vi "test-0mq.vi"() -> ()   [LabVIEW 2020]
uses:
  <vilib>/addons/zeromq/socket_type.ctl
  <vilib>/addons/zeromq/zmq_context.lvclass
  <vilib>/addons/zeromq/zeromq.lvlib
  <vilib>/addons/zeromq/zmq_socket.lvclass
panel:
  out "?":string
  in  "stop":bool
  out "error out":errorcluster
  out "data":string
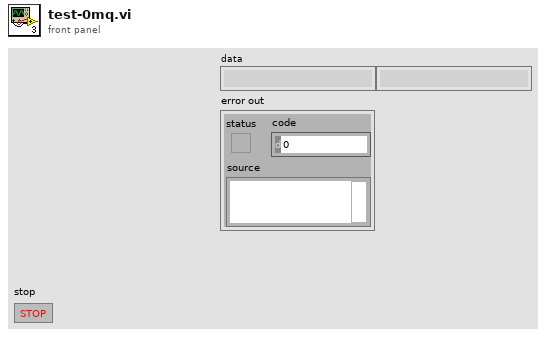
[diagram p1: front panel]
types:
  T1 = typedef "zeromq.lvlib/socket_type.ctl" = enum8{"ZMQ_PAIR", "ZMQ_PUB", "ZMQ_SUB", "ZMQ_REQ", "ZMQ_REP", "ZMQ_DEALER", "ZMQ_ROUTER", "ZMQ_PULL", "ZMQ_PUSH", "ZMQ_XPUB", "ZMQ_XSUB", "ZMQ_STREAM", "ZMQ_SERVER", "ZMQ_CLIENT", "ZMQ_RADIO", "ZMQ_DISH", "ZMQ_GATHER", "ZMQ_SCATTER", "ZMQ_DGRAM"}
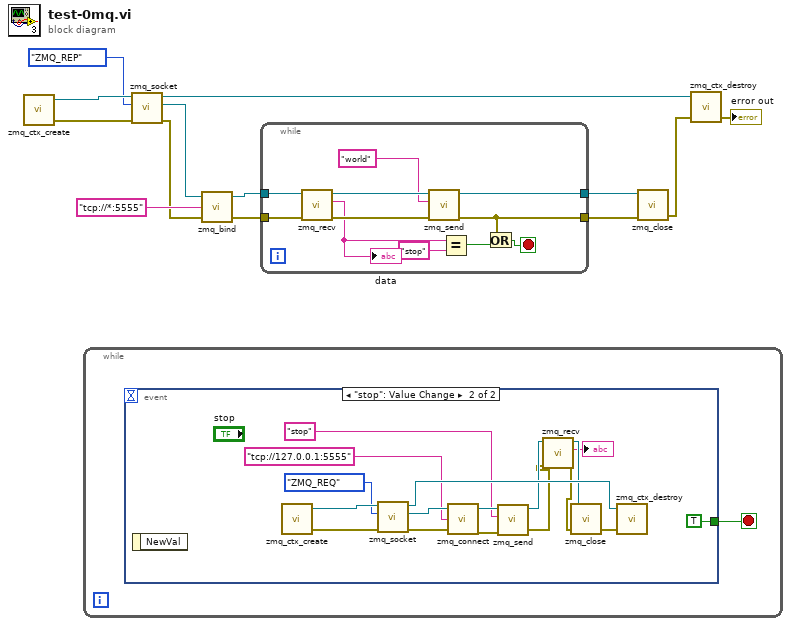
[diagram p0: block diagram]
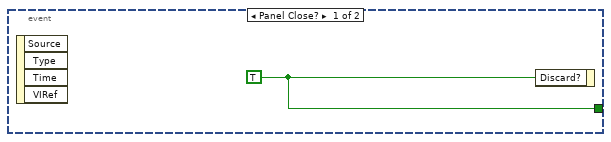
[diagram p2: hidden frame]
diagram:
  n1 = call <vilib>:"zmq_ctx_create.vi"() -> ("error out"=w12:errorcluster, "context out"=w13:refnum<class "zmq_context.lvclass">)  [unwired: 4 in]
  n2 = while {
    stop <- w14 stop-if-true
    n3 = event shown="[1] \"stop\": Value Change" {
      selector: _ -> [_ _]
      dyn-events: _ -> [_ _]
      timeout: _ -> [_ _]
      tunnel: [w15 TRUE] -> w14
      event Panel Close? {
        w15 = TRUE
        n4 = event-data() -> ()  [unwired: 1 in, 4 out]
        n5 = event-data("Discard?"=w15) -> ()  [unwired: 1 in, 1 out]
      }
      event "stop": Value Change {
        n6 = event-data() -> ()  [unwired: 1 in, 1 out]
        n7 = call <vilib>:"zmq_ctx_create.vi"() -> ("error out"=w26:errorcluster, "context out"=w25:refnum<class "zmq_context.lvclass">)  [unwired: 4 in]
        n8 = call <vilib>:"zmq_socket.vi"("error in"=w26, "socket type"=socket_type."ZMQ_REQ", "context in"=w25) -> ("error out"=w28:errorcluster, "socket out"=w27:refnum<class "zmq_socket.lvclass">, "context out"=w32:refnum<class "zmq_context.lvclass">)  [unwired: 2 in]
        n9 = call <vilib>:"zmq_connect.vi"("error in"=w28, "endpoint"="tcp://127.0.0.1:5555", "socket in"=w27) -> ("error out"=w30:errorcluster, "socket out"=w29:refnum<class "zmq_socket.lvclass">)  [unwired: 1 in]
        n10 = call <vilib>:"zmq_send.vi"("error in"=w30, "data"="stop", "socket in"=w29) -> ("error out"=w19:errorcluster, "socket out"=w20:refnum<class "zmq_socket.lvclass">)  [unwired: 4 in]
        n11 = call <vilib>:"zmq_recv.vi"("error in"=w19, "socket in"=w20) -> ("error out"=w17:errorcluster, "data"=→"?":string, "socket out"=w18:refnum<class "zmq_socket.lvclass">)  [unwired: 3 in, 2 out]
        n12 = call <vilib>:"zmq_close.vi"("error in"=w17, "socket"=w18) -> ("error out"=w31:errorcluster)  [unwired: 3 in]
        n13 = call <vilib>:"zmq_ctx_destroy.vi"("error in"=w31, "context in"=w32) -> ()  [unwired: 3 in, 1 out]
      }
    }
  }
  n14 = call <vilib>:"zmq_socket.vi"("error in"=w12, "socket type"=socket_type."ZMQ_REP", "context in"=w13) -> ("error out"=w7:errorcluster, "socket out"=w9:refnum<class "zmq_socket.lvclass">, "context out"=w10:refnum<class "zmq_context.lvclass">)  [unwired: 2 in]
  n15 = call <vilib>:"zmq_bind.vi"("error in"=w7, "endpoint"="tcp://*:5555", "socket in"=w9) -> ("error out"=w5:errorcluster, "socket out"=w6:refnum<class "zmq_socket.lvclass">)  [unwired: 1 in]
  n16 = while {
    tunnel: w6 -> [w43]
    tunnel: w5 -> [w42]
    tunnel: [w39] -> w4
    tunnel: [w37] -> w3
    stop <- w34 stop-if-true
    n17 = call <vilib>:"zmq_recv.vi"("error in"=w42, "socket in"=w43) -> ("error out"=w40:errorcluster, "data"=w36:string, "socket out"=w41:refnum<class "zmq_socket.lvclass">)  [unwired: 3 in, 2 out]
    "data" <- w36
    n18 = call <vilib>:"zmq_send.vi"("error in"=w40, "data"="world", "socket in"=w41) -> ("error out"=w37:errorcluster, "socket out"=w39:refnum<class "zmq_socket.lvclass">)  [unwired: 4 in]
    n19 = Equal?(x=w36, y="stop") -> (x = y?=w33:bool)
    n20 = Or(x=w37, y=w33) -> (x .or. y?=w34:bool)
  }
  n21 = call <vilib>:"zmq_close.vi"("error in"=w3, "socket"=w4) -> ("error out"=w2:errorcluster)  [unwired: 3 in]
  n22 = call <vilib>:"zmq_ctx_destroy.vi"("error in"=w2, "context in"=w10) -> ("error out"=→"error out":errorcluster)  [unwired: 3 in]
